vi "bad1.vi"() -> ()   [LabVIEW 2013]
uses:
  <vilib>/NI/Tag Bus/table/data table.ctl
  <vilib>/NI/Tag Bus/table/transfer specification.ctl
  <vilib>/NI/Tag Bus/tag/Data Type.ctl
  <vilib>/Platform/TimedLoop/XDataNode/timing_clust.ctl
  <vilib>/Platform/TimedLoop/XDataNode/nitl_modes.ctl
  <vilib>/Platform/TimedLoop/XDataNode/wakeup.ctl
  <vilib>/platform/TimedLoop/XDataNode/XDataNode.xnode
  <vilib>/NI/Tag Bus/table/data table.lvlib
  <vilib>/Platform/TimedLoop/XDataNode/XDNodeRunTimeDep.lvlib
  <vilib>/NI/Tag Bus/tag/tag descriptor.lvclass
panel:
  out "input data":T1
  out "data table sink out":T1
  out "error out":errorcluster
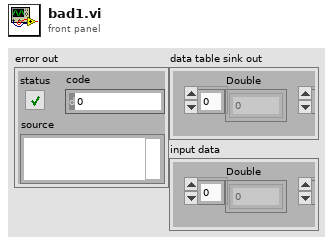
[diagram p1: front panel]
types:
  T1 = typedef "tag bus.lvlib/data table.lvlib/data table.ctl" = cluster{"Double":dbl[], "Single":sgl[], "I64":i64[], "I32":i32[], "I16":i16[], "I8":i8[], "U64":u64[], "U32":u32[], "U16":u16[], "U8":u8[], "Boolean":bool[], "String":string[], "Array of Double":cluster{"DBL Array":dbl[]}[], "Array of Single":cluster{"SGL Array":sgl[]}[], "Array of I64":cluster{"I64 Array":i64[]}[], "Array of I32":cluster{"I32 Array":i32[]}[], "Array of I16":cluster{"I16 Array":i16[]}[], "Array of I8":cluster{"I8 Array":i8[]}[], "Array of U64":cluster{"U64 Array":u64[]}[], "Array of U32":cluster{"U32 Array":u32[]}[], "Array of U16":cluster{"U16 Array":u16[]}[], "Array of U8":cluster{"U8 Array":u8[]}[], "Array of Boolean":cluster{"Boolean Array":bool[]}[], "Array of String":cluster{"String Array":string[]}[]}
  T2 = typedef "tag bus.lvlib/tag descriptor.lvclass/Data Type.ctl" = enum16{"Double", "Single", "I64", "I32", "I16", "I8", "U64", "U32", "U16", "U8", "Boolean", "String", "Array of Double", "Array of Single", "Array of I64", "Array of I32", "Array of I16", "Array of I8", "Array of U64", "Array of U32", "Array of U16", "Array of U8", "Array of Boolean", "Array of String"}
  T3 = typedef "tag bus.lvlib/data table.lvlib/transfer specification.ctl" = cluster{"data type":T2, "sink indices":i32[], "source indices":i32[]}
  T4 = typedef "XDNodeRunTimeDep.lvlib/timing_clust.ctl" = cluster{"Expected End [f-1]":u64, "Actual End [f-1]":u64, "Finished Late? [f-1]":bool, "Expected End [i-1]":u64, "Actual End [i-1]":u64, "Finished Late? [i-1]":bool, "Expected Start [i]":u64, "Actual Start [i]":u64, "Expected Start [f]":u64, "Actual Start [f]":u64, "Source Name":string, "Structure Name":string, "Period":i64, "Deadline":i64, "Offset":i64, "Start":i64, "Priority":i32, "Timeout":i32, "Mode":T5, "Wakeup Reason":T6, "Error":errorcluster, "Source Type":string, "Secondary Source Type":string, "Global End Time":u64, "Global Start Time":u64, "Frame Duration":u64, "Iteration Duration":u64, "Assigned CPU":i32, "I/O Scan Engine Mode":u32}
  T5 = typedef "XDNodeRunTimeDep.lvlib/nitl_modes.ctl" = enum32{"No Change", "Process missed periods, maintain original phase", "Discard missed periods, maintain original phase", "Process missed periods, ignore original phase", "Discard missed periods, ignore original phase"}
  T6 = typedef "XDNodeRunTimeDep.lvlib/wakeup.ctl" = enum32{"Normal", "Aborted", "Asynchronous wakeup", "Timing source error", "Timed loop error", "Timeout"}
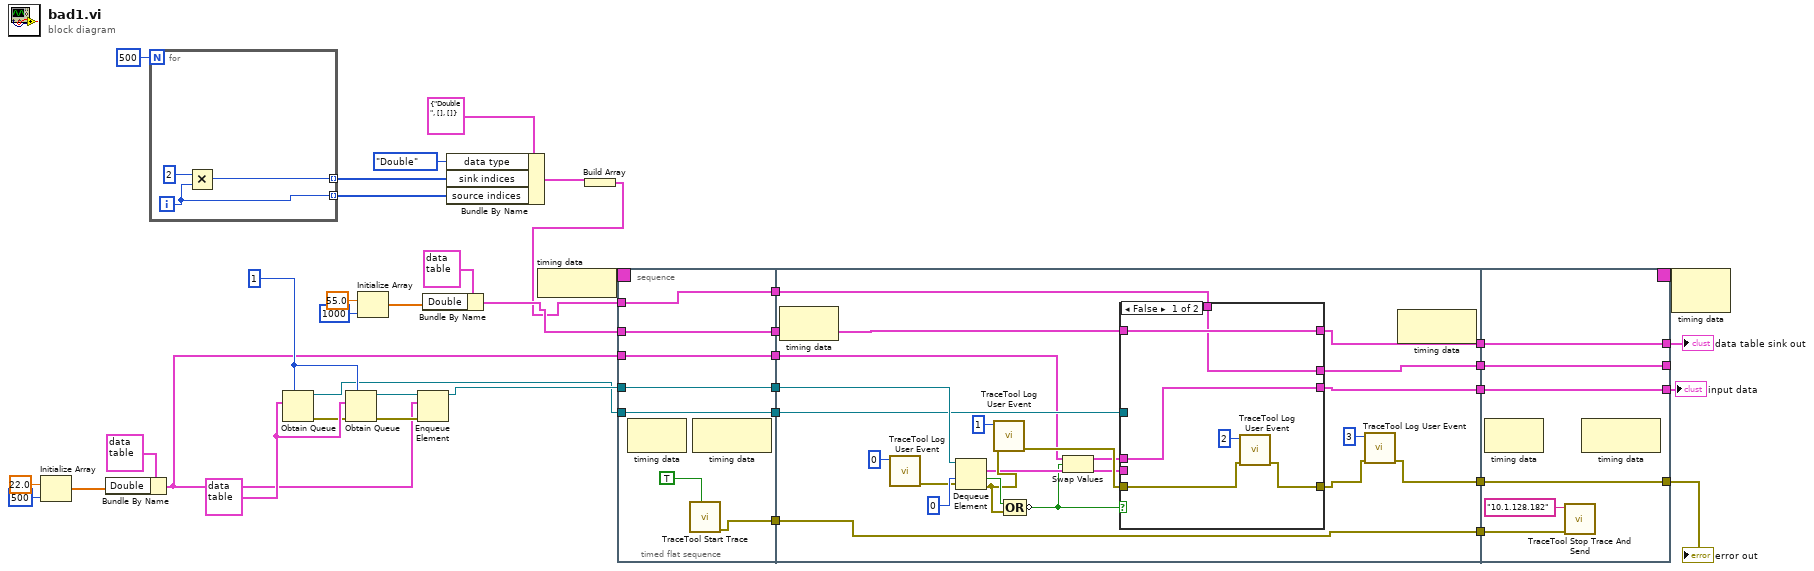
[diagram p0: block diagram]
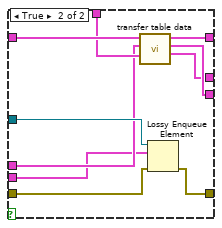
[diagram p2: hidden frame]
diagram:
  w28 = 1 ("max queue size (-1, unlimited)")
  w29 = T1 {"Double"=[], "Single"=[], "I64"=[], "I32"=[], "I16"=[], "I8"=[], "U64"=[], "U32"=[], "U16"=[], "U8"=[], "Boolean"=[], "String"=[], "Array of Double"=[], "Array of Single"=[], "Array of I64"=[], "Array of I32"=[], "Array of I16"=[], "Array of I8"=[], "Array of U64"=[], "Array of U32"=[], "Array of U16"=[], "Array of U8"=[], "Array of Boolean"=[], "Array of String"=[]} ("input data")
  n1 = Initialize Array(22.0 ("element"), 500 ("dimension size")) -> (w21:dbl[])
  n2 = Bundle By Name(cluster=T1 {"Double"=[], "Single"=[], "I64"=[], "I32"=[], "I16"=[], "I8"=[], "U64"=[], "U32"=[], "U16"=[], "U8"=[], "Boolean"=[], "String"=[], "Array of Double"=[], "Array of Single"=[], "Array of I64"=[], "Array of I32"=[], "Array of I16"=[], "Array of I8"=[], "Array of U64"=[], "Array of U32"=[], "Array of U16"=[], "Array of U8"=[], "Array of Boolean"=[], "Array of String"=[]} ("input data"), "Double"=w21) -> (w11:T1)
  n3 = for {
    N: 500 -> [_]
    tunnel: [w31] -> w6 mode=indexing
    tunnel: [w30] -> w5 mode=indexing
    i -> [w30]
    n4 = Multiply(x=2, y=w30) -> (x*y=w31:i32)
  }
  n5 = Obtain Queue(max queue size (-1, unlimited)=w28, element data type=w29) -> (queue out=w1:refnum<queue>, error out=w25:errorcluster)  [unwired: 3 in, 1 out]
  n6 = Obtain Queue(max queue size (-1, unlimited)=w28, element data type=w29, error in (no error)=w25) -> (queue out=w23:refnum<queue>, error out=w24:errorcluster)  [unwired: 2 in, 1 out]
  n7 = Initialize Array(55.0 ("element"), 1000 ("dimension size")) -> (w16:dbl[])
  n8 = Enqueue Element(queue=w23, element=w11, error in (no error)=w24) -> (queue out=w2:refnum<queue>)  [unwired: 1 in, 2 out]
  n9 = Bundle By Name(cluster=T1 {"Double"=[], "Single"=[], "I64"=[], "I32"=[], "I16"=[], "I8"=[], "U64"=[], "U32"=[], "U16"=[], "U8"=[], "Boolean"=[], "String"=[], "Array of Double"=[], "Array of Single"=[], "Array of I64"=[], "Array of I32"=[], "Array of I16"=[], "Array of I8"=[], "Array of U64"=[], "Array of U32"=[], "Array of U16"=[], "Array of U8"=[], "Array of Boolean"=[], "Array of String"=[]} ("input data"), "Double"=w16) -> (w13:T1)
  n10 = Bundle By Name(cluster=T3 {"data type"=enum."Double", "sink indices"=[], "source indices"=[]} ("merge specification"), "data type"=Data_Type."Double", "sink indices"=w6, "source indices"=w5) -> (w7:T3)
  n11 = node-c288() -> (w27:T4)
  n12 = Build Array(w7) -> (w3:T3[])
  n13 = timed-sequence {
    timing: w27 -> [_]
    timing-out: [_] -> w26
    tunnel: w2 -> [w52]
    tunnel: w1 -> [w51]
    tunnel: [w50] -> w15
    tunnel: w13 -> [w49]
    tunnel: [w48] -> w12
    tunnel: w11 -> [w47]
    tunnel: [w46] -> w10
    tunnel: [w45] -> _
    tunnel: w3 -> [w34]
    n14 = timed-flat-sequence {
      tunnel: w47 -> [w56]
      tunnel: w49 -> [w57]
      tunnel: w51 -> [w58]
      tunnel: w52 -> [w59]
      tunnel: [w59] -> w40
      tunnel: [w58] -> w39
      tunnel: [w57] -> w38
      tunnel: [w56] -> w37
      tunnel: [w54] -> w36
      tunnel: w34 -> [w53]
      tunnel: [w53] -> w33
      tunnel: [w67] -> w44
      tunnel: [w79] -> w43
      tunnel: [w78] -> w42
      tunnel: [w77] -> w41
      tunnel: w40 -> [w82]
      tunnel: w39 -> [w81]
      tunnel: w38 -> [w80]
      tunnel: w37 -> [w66]
      tunnel: w36 -> [w76]
      tunnel: [w76] -> w35
      tunnel: w33 -> [w71]
      tunnel: [w105] -> w45
      tunnel: [w106] -> w46
      tunnel: [w107] -> w48
      tunnel: [w108] -> w50
      tunnel: w44 -> [w108]
      tunnel: w43 -> [w107]
      tunnel: w42 -> [w106]
      tunnel: w41 -> [w105]
      tunnel: w35 -> [w104]
      frame #0 {
        n15 = node-c288() -> ()  [unwired: 1 in, 1 out]
        n16 = call <vilib>:"TraceTool Start Trace.vi"("Detailed Tracing? (F)"=TRUE) -> ("error out"=w54:errorcluster)  [unwired: 9 in, 1 out]
        n17 = node-c288() -> ()  [unwired: 1 in, 1 out]
      }
      frame #1 {
        n18 = node-c288() -> ()  [unwired: 1 in, 1 out]
        n19 = call <vilib>:"TraceTool Log User Event.vi"("Event ID (0-255)"=u32 0) -> ("error out"=w72:errorcluster)  [unwired: 10 in]
        n20 = Dequeue Element(queue=w82, timeout in ms (-1)=0, error in (no error)=w72) -> (element=w65:T1, timed out?=w84:bool, error out=w69:errorcluster)  [unwired: 1 out]
        n21 = call <vilib>:"TraceTool Log User Event.vi"("error in (no error)"=w69, "Event ID (0-255)"=u32 1) -> ("error out"=w68:errorcluster)  [unwired: 9 in]
        n22 = Compound Arithmetic op=OR(w84, w69) -> (invert w64:bool)
        n23 = Swap Values(12:w66, 13:w64, 14:w65) -> (1:w63:T1, 3:w62:T1)
        n24 = case shown="False" w64 {
          tunnel: [w90 w100] -> w79
          tunnel: [w85 w99] -> w78
          tunnel: [w89 w98] -> w77
          tunnel: w68 -> [w87 w97]
          tunnel: [w86 w96] -> w70
          tunnel: w81 -> [_ w95]
          tunnel: w80 -> [w90 w94]
          tunnel: w71 -> [w89 w93]
          tunnel: w63 -> [w85 w92]
          tunnel: w62 -> [_ w91]
          frame False {
            n25 = call <vilib>:"TraceTool Log User Event.vi"("error in (no error)"=w87, "Event ID (0-255)"=u32 2) -> ("error out"=w86:errorcluster)  [unwired: 9 in]
          }
          frame True {
            n26 = call <vilib>:"transfer table data.vi"("transfer specification in"=w93, "data table source in"=w92, "data table sink in"=w94) -> ("transfer specification out"=w98:T3[], "data table source out"=w99:T1, "data table sink out"=w100:T1)  [unwired: 6 in]
            n27 = Lossy Enqueue Element(queue=w95, element=w91, error in (no error)=w97) -> (error out=w96:errorcluster)  [unwired: 3 out]
          }
        }
        n28 = call <vilib>:"TraceTool Log User Event.vi"("error in (no error)"=w70, "Event ID (0-255)"=u32 3) -> ("error out"=w67:errorcluster)  [unwired: 9 in]
        n29 = node-c288() -> ()  [unwired: 1 in, 1 out]
      }
      frame #2 {
        n30 = node-c288() -> ()  [unwired: 1 in, 1 out]
        n31 = call <vilib>:"TraceTool Stop Trace And Send.vi"("error in (no error)"=w104, "Trace Host Network Address"="10.1.128.182") -> ()  [unwired: 9 in, 1 out]
        n32 = node-c288() -> ()  [unwired: 1 in, 1 out]
      }
    }
  }
  "error out" <- w15
  "data table sink out" <- w12
  "input data" <- w10
  n33 = node-c288(w26) -> ()  [unwired: 1 out]
